vi "AES Data Replay Voltage Scaling.vi"(4 "output value below threshold speed (0)":i16, 6 "APU.Degrees per Tick":fxp<+/-,47,-4>, 7 "negate voltage when speed negative?":bool, 8 "speed threshold":fxp<+/-,47,-4>, 9 "voltage scaling intercept":fxp<+/-,18,3>, 10 "voltage scaling slope":fxp<+,18,12>, 11 "replay data":i16) -> (3 "output value":i16)   [LabVIEW 2010, in "AES.lvlib" / "AES FPGA.lvlib"]
doc: "Uses the provided slope (m) and intercept (b) to compute a voltage scaler that is based upon APU speed. This scale factor is used upon the replay data to generate the output value. Additionally, if the APU speed is less than or equal to the speed threshold, the output value below threshold is used instead.\n\nIf (APU.Degrees per tick >= speed threshold)\n output value = (m * APU.Degrees per tick + b) * replay data\nelse\n output value = output value below threshold\n\nAdditionally, the output value will be negated if engine speed is negative and \"negate voltage when speed negative?\" is true. This is useful for VR sensor playback in reverse engine speed situations."
uses:
  AES FPGA.lvlib
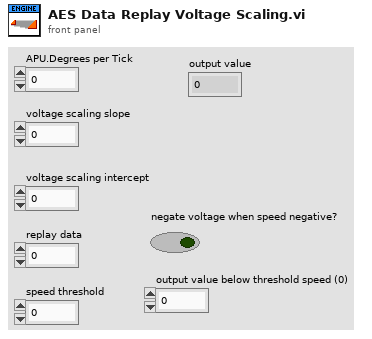
[diagram p1: front panel]
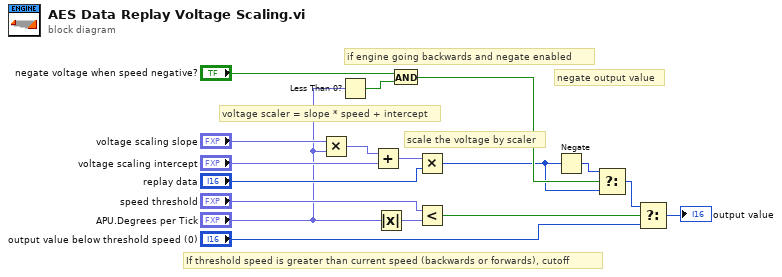
[diagram p0: block diagram]
diagram:
  # "if engine going backwards and negate enabled"
  # "negate output value"
  # "If threshold speed is greater than current speed (backwards or forwards), cutoff"
  # "scale the voltage by scaler"
  # "voltage scaler = slope * speed + intercept"
  n1 = Multiply(x="voltage scaling slope", y="APU.Degrees per Tick") -> (x*y=w13:fxp<+/-,25,4>)
  n2 = Less Than 0?(x="APU.Degrees per Tick") -> (x < 0?=w7:bool)
  n3 = Add(x=w13, y="voltage scaling intercept") -> (x+y=w16:fxp<+/-,25,4>)
  n4 = Absolute Value(x="APU.Degrees per Tick") -> (abs(x)=w9:fxp<+,47,-4>)
  n5 = And(x="negate voltage when speed negative?", y=w7) -> (x .and. y?=w4:bool)
  n6 = Multiply(x=w16, y="replay data") -> (x*y=w3:i16)
  n7 = Less?(x="speed threshold", y=w9) -> (x < y?=w12:bool)
  n8 = Negate(x=w3) -> (-x=w5:i16)
  n9 = Select(t=w5, s=w4, f=w3) -> (s? t:f=w2:i16)
  n10 = Select(t=w2, s=w12, f="output value below threshold speed (0)") -> (s? t:f=→"output value":i16)
